vi "First Run Check.vi"() -> (8 "First Run?":bool)   [LabVIEW 2014]
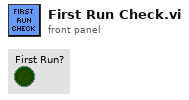
[diagram p1: front panel]
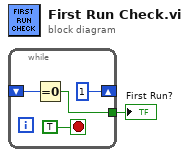
[diagram p0: block diagram]
diagram:
  n1 = while {
    shift-right: [u8 1] -> _
    shift-left: _ -> [w3]
    tunnel: [w2] -> w1
    stop <- TRUE stop-if-true
    n2 = Equal To 0?(x=w3) -> (x = 0?=w2:bool)
  }
  "First Run?" <- w1
